vi "Add SRs.vi"(8 "error in":errorcluster, 9 "entered SRs in":i32[](array[numeric]), 11 "Data Loop Data in":T1) -> (0 "error out":errorcluster, 3 "Data Loop Data out":T1)   [LabVIEW 2018]
uses:
  Type Defs/Data Loop Data.ctl
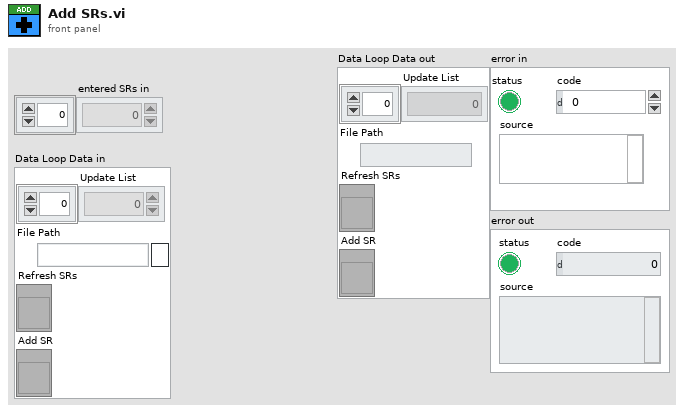
[diagram p1: front panel]
types:
  T1 = typedef "Data Loop Data.ctl" = cluster{"Update List":i32[], "File Path":path, "Refresh SRs":refnum<vi>, "Add SR":refnum<vi>}
  T2 = typedef "SR Cluster.ctl" = cluster{"Color":u32, "SR Number":i32, "SR Status":T3, "Name":string, "Summary":string, "Last Updated":timestamp, "SR Type":string, "Service Level":string, "Days Open":dbl, "Creation Date":timestamp}
  T3 = typedef "SR Status.ctl" = enum16{"Caller Abandoned", "Created in Error", "Expired", "Forum Resolved AE", "Forum Resolved Customer", "IN WORK", "IN WORK Collab with AES", "IN WORK Collab with PSE", "IN WORK Collab with SE", "IN WORK Customer Added Note", "IN WORK Escalation", "IN WORK Wait on Customer", "Open", "Potentially Resolved", "Presumed Resolved", "RMA Approved for Return", "Resolved", "Passed Off"}
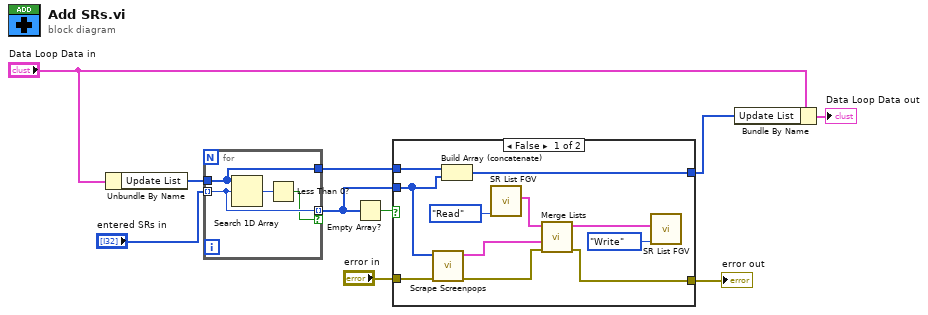
[diagram p0: block diagram]
diagram:
  n1 = Unbundle By Name("Data Loop Data in") -> ("Update List"=w10:i32[])
  n2 = for {
    tunnel: "entered SRs in" -> [w13] mode=indexing
    tunnel: w10 -> [w11]
    tunnel: [w13] -> w5 mode=indexing if=w12
    tunnel: [w11] -> w4
    n3 = Search 1D Array(1D array=w11, element=w13) -> (index of element=w14:i32)  [unwired: 1 in]
    n4 = Less Than 0?(x=w14) -> (x < 0?=w12:bool)
  }
  n5 = Empty Array?(array=w5) -> (empty?=w6:bool)
  n6 = case shown="False" w6 {
    tunnel: w5 -> [w21 _]
    tunnel: [w22 w27] -> w3
    tunnel: w4 -> [w25 w27]
    tunnel: "error in" -> [w20 w26]
    tunnel: [w18 w26] -> w1
    frame False {
      n7 = call "Scrape Screenpops.vi"("error in"=w20, "SR number list in"=w21) -> ("error out"=w19:errorcluster, "sr clusters out"=w17:T2[])  [unwired: 8 in]
      n8 = Build Array (concatenate)(w25, w21) -> (w22:i32[])
      n9 = call "SR List FGV.vi"("Operation"=enum16{"Initialize", "Write", "Read", "Clear"}."Read") -> ("list out"=w24:T2[])  [unwired: 9 in, 1 out]
      n10 = call "Merge Lists.vi"("error in"=w19, "new list in"=w17, "list in"=w24) -> ("error out"=w18:errorcluster, "list out"=w15:T2[])  [unwired: 7 in]
      n11 = call "SR List FGV.vi"("Operation"=enum16{"Initialize", "Write", "Read", "Clear"}."Write", "list in"=w15) -> ()  [unwired: 8 in, 2 out]
    }
    frame True {
    }
  }
  "error out" <- w1
  n12 = Bundle By Name(cluster="Data Loop Data in", "Update List"=w3) -> (→"Data Loop Data out":T1)
